vi "RSZVL_MeasPwrAtFreq.vi"(0 "VISA resource name":refnum<visa-resource-name>, 1 "Route Names":string[](array[string]), 5 "Center Frequency (100MHz)":dbl=1000000000.0 format="%^.3e", 7 "Span Frequency (50 kHz)":dbl=50000.0, 9 "Frequency to meas PWR At":dbl, 11 "error in (no error)":errorcluster {"code" format="%.0x"}, 12 "Reference Level (-20.0)":dbl=-20.0 format="%^.3e", 13 "Calibration Enabled":bool) -> (3 "Marker Position":dbl format="%^.3e", 4 "VISA resource name out":refnum<visa-resource-name>, 6 "Marker Amplitude":dbl caption="Marker Amplitude (raw)" format="%^.3e", 10 "Marker Amplitude (Cal)":dbl, 15 "error out":errorcluster {"code" format="%.0x"})   [LabVIEW 2015]
doc: "This VI performs:\n1- Setup Center Frequency and Span Frequency \n2- Setup Reference Level (Max -10dBm)\n3- Enable Marker at the Specified Frequency (if 0, uses Center Frequency)\n4- Reads Marker (Power at the specified Frequency)\n5- Adjust measurement for path losses (Calibration)"
uses:
  <vilib>/ErrorRing/Error Ring.xnode
  <vilib>/Utility/error.llb/Error Cluster From Error Code.vi
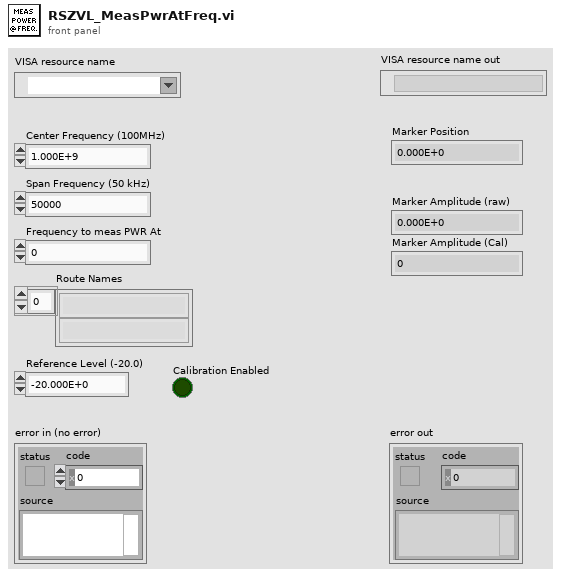
[diagram p1: front panel]
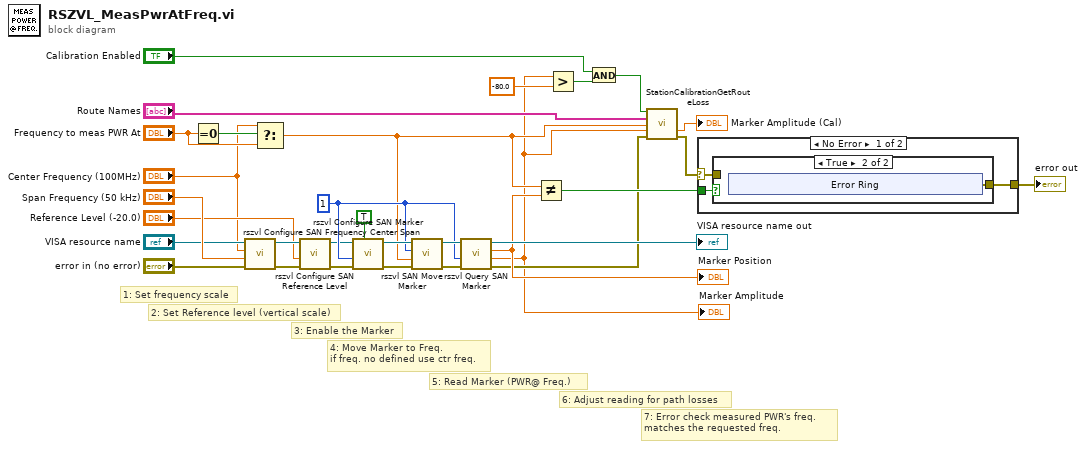
[diagram p0: block diagram]
diagram:
  w29 = 1 ("Marker (1)")
  # "7: Error check measured PWR's freq. \nmatches the requested freq."
  # "2: Set Reference level (vertical scale)"
  # "6: Adjust reading for path losses"
  # "5: Read Marker (PWR@ Freq.)"
  # "4: Move Marker to Freq.\nif freq. no defined use ctr freq."
  # "3: Enable the Marker"
  # "1: Set frequency scale"
  n1 = Equal To 0?(x="Frequency to meas PWR At") -> (x = 0?=w15:bool)
  n2 = call <instrlib>:"rszvl Configure SAN Frequency Center Span.vi"("error in (no error)"="error in (no error)", "Span"="Span Frequency (50 kHz)", "Center Frequency"="Center Frequency (100MHz)", "VISA resource name"="VISA resource name") -> ("error out"=w17:errorcluster, "VISA resource name out"=w20:refnum<visa-resource-name>)  [unwired: 6 in]
  n3 = Select(t="Center Frequency (100MHz)", s=w15, f="Frequency to meas PWR At") -> (s? t:f=w8:dbl)
  n4 = call <instrlib>:"rszvl Configure SAN Reference Level.vi"("error in (no error)"=w17, "Reference Level (-20.0)"="Reference Level (-20.0)", "VISA resource name"=w20) -> ("error out"=w18:errorcluster, "VISA resource name out"=w19:refnum<visa-resource-name>)  [unwired: 7 in]
  n5 = call <instrlib>:"rszvl Configure SAN Marker.vi"("Marker Enabled (Off)"=TRUE, "error in (no error)"=w18, "Marker (1)"=w29, "VISA resource name"=w19) -> ("error out"=w28:errorcluster, "VISA resource name out"=w31:refnum<visa-resource-name>)  [unwired: 6 in]
  n6 = call <instrlib>:"rszvl SAN Move Marker.vi"("error in (no error)"=w28, "Marker Position (0.0)"=w8, "Marker (1)"=w29, "VISA resource name"=w31) -> ("error out"=w27:errorcluster, "VISA resource name out"=w30:refnum<visa-resource-name>)  [unwired: 6 in]
  n7 = call <instrlib>:"rszvl Query SAN Marker.vi"("error in (no error)"=w27, "Marker (1)"=w29, "VISA resource name"=w30) -> ("error out"=w7:errorcluster, "Marker Amplitude"=w4:dbl, "Marker Position"=w12:dbl, "VISA resource name out"=→"VISA resource name out":refnum<visa-resource-name>)  [unwired: 5 in]
  "Marker Position" <- w12
  "Marker Amplitude" <- w4
  n8 = Not Equal?(x=w8, y=w12) -> (x != y?=w11:bool)
  n9 = Greater?(x=w4, y=-80.0) -> (0:w3:bool)
  n10 = And(x="Calibration Enabled", y=w3) -> (x .and. y?=w1:bool)
  n11 = call "StationCalibrationGetRouteLoss.vi"("Calibration Enabled"=w1, "Route Names"="Route Names", "Frequency"=w8, "Power Level"=w4, "error in (no error)"=w7) -> ("Adjusted Power Level"=→"Marker Amplitude (Cal)":dbl, "error out"=w5:errorcluster)  [unwired: 7 in, 2 out]
  n12 = case shown="No Error" w5 {
    selector: w5 -> [w32 w42]
    tunnel: w11 -> [w34 _]
    tunnel: [w33 w42] -> w10
    frame No Error {
      n13 = case shown="True" w34 {
        tunnel: [w35 w36] -> w33
        tunnel: w32 -> [w35 _]
        frame False {
        }
        frame True {
          n14 = xnode "Error Ring"() -> ("error out"=w36:errorcluster)
        }
      }
    }
    frame Error {
    }
  }
  "error out" <- w10
